vi "Begin.vi"(8 "error in":errorcluster) -> (0 "error out":errorcluster)   [LabVIEW 2018]
doc: "Called before other user functions, this VI is expected to open initial I/O refnums, load in file data, and do all program initialization. Notice that the <B>error out</B> terminal is simply used for data flow. Wiring it to other structures or subVIs ensures that this VI runs first."
uses:
  <vilib>/Rock Robotics/SystemInterfaces/DIO/FPGA_DIOPWMChannel.ctl
  <vilib>/Rock Robotics/WPI/SafetyOutput/WPI_SafetyOutputConfigMenu.ctl
  <vilib>/Rock Robotics/WPI/DriverStation/WPI_DriverStationRobotMode2.ctl
  <vilib>/Rock Robotics/WPI/Joystick/WPI_JoystickDeviceEnum.ctl
  <vilib>/Rock Robotics/WPI/Solenoid/WPI_SolenoidChannel.ctl
  <vilib>/Rock Robotics/WPI/Accelerometer/WPI_AccelerometerRange.ctl
  <vilib>/Rock Robotics/SystemInterfaces/DIO/FPGA_DIOChannel.ctl
  <vilib>/Rock Robotics/WPI/RobotDrive/WPI_RobotDriveOpen2MotorWithSPARK.vi
  Robot Global Data.vi
  <vilib>/Rock Robotics/Network Tables/NT Write String Array.vi
  <vilib>/Rock Robotics/WPI/Solenoid/WPI_SolenoidOpenSingle.vi
  <vilib>/Rock Robotics/WPI/Accelerometer/InternalAccelerometer/WPI_AccelerometerInternalOpen.vi
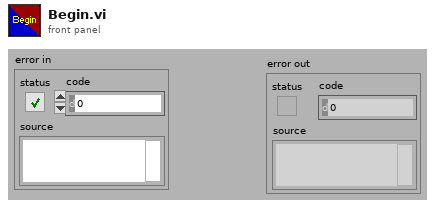
[diagram p1: front panel]
types:
  T1 = typedef "FPGA_DIOChannel.ctl" = enum8{"DIO 0", "DIO 1", "DIO 2", "DIO 3", "DIO 4", "DIO 5", "DIO 6", "DIO 7", "DIO 8", "DIO 9", "DIO MXP 0", "DIO MXP 1", "DIO MXP 2", "DIO MXP 3", "DIO MXP 4", "DIO MXP 5", "DIO MXP 6", "DIO MXP 7", "DIO MXP 8", "DIO MXP 9", "DIO MXP 10", "DIO MXP 11", "DIO MXP 12", "DIO MXP 13", "DIO MXP 14", "DIO MXP 15", "SPI Port CS1", "SPI Port CS2", "SPI Port CS3", "SPI Port MISO", "SPI Port MOSI", "Invalid"}
  T2 = typedef "WPI_SolenoidChannel.ctl" = enum8{"Solenoid 0", "Solenoid 1", "Solenoid 2", "Solenoid 3", "Solenoid 4", "Solenoid 5", "Solenoid 6", "Solenoid 7", "Invalid"}
  T3 = typedef "WPI_AccelerometerRange.ctl" = enum16{"+/- 2 g", "+/- 4 g", "+/- 8 g"}
  T4 = typedef "WPI_JoystickDeviceEnum.ctl" = enum16{"USB 0", "USB 1", "USB 2", "USB 3", "USB 4", "USB 5"}
  T5 = typedef "WPI_DriverStationRobotMode2.ctl" = enum16{"Autonomous Disabled", "Autonomous Enabled", "Teleop Disabled", "Teleop Enabled", "Disconnected", "Finish", "Test Disabled", "Test Enabled", "Emergency Stopped"}
  T6 = typedef "WPI_SafetyOutputConfigMenu.ctl" = enum16{"Enable", "Disable"}
  T7 = typedef "FPGA_DIOPWMChannel.ctl" = enum8{"PWM 0", "PWM 1", "PWM 2", "PWM 3", "PWM 4", "PWM 5", "PWM 6", "PWM 7", "PWM 8", "PWM 9", "PWM MXP 0", "PWM MXP 1", "PWM MXP 2", "PWM MXP 3", "PWM MXP 4", "PWM MXP 5", "PWM MXP 6", "PWM MXP 7", "PWM MXP 8", "PWM MXP 9", "Invalid"}
  T8 = typedef "WPI_JoystickDevRef.ctl" = cluster{"Device":T4}
  T9 = typedef "WPI_RobotDriveDevRef.ctl" = cluster{"DevStatus":errorcluster, "Motors[]":T10[], "Square Inputs":bool, "Max Output":dbl}
  T10 = typedef "WPI_MotorControlDeviceRef.ctl" = cluster{"DeviceStatus":errorcluster, "Type":T11, "PWM":cluster{"PWM Channel":T7, "DeadBand":T12}, "CAN":cluster{"Device Number":u8, "SetOutput VI Ref":variant, "GetOutput VI Ref":variant, "Enable VI Ref":variant, "Disable VI Ref":variant, "Data":variant}, "Invert":bool, "DIO PWM":cluster{"PWM \"Enable\" Channel":T7, "DIOChannel":T1, "PWM Rate":dbl}}
  T11 = typedef "WPI_MotorControlType.ctl" = enum16{"PWM", "CAN", "DIO PWM"}
  T12 = typedef "WPI_PWMDeadband.ctl" = cluster{"Name":string, "maxPositivePwm":i32, "minPositivePwm":i32, "centerPwm":i32, "maxNegativePwm":i32, "minNegativePwm":i32, "angularRange":u16}
  T13 = typedef "WPI_AccelerometerDevRef.ctl" = cluster{"DevStatus":errorcluster, "Scaling":T14, "Analog Channels":T15, "I2C Bus":T17, "SPI Bus":T18, "Accel Range":T19, "ADXL Axes":T20, "Handle":i32, "Device Address":u8, "Accel Type":enum16{"Analog", "ADXL345 I2C", "ADXL345 SPI", "Internal", "ADXL362 SPI"}}
  T14 = typedef "WPI_AccelerometerScaling.ctl" = cluster{"Gain (VoltsPerG)":dbl, "Center Voltage":dbl}
  T15 = typedef "WPI_AccelerometerAnalogChannels.ctl" = cluster{"X-Axis":T16, "Y-Axis":T16, "Z-Axis":T16}
  T16 = typedef "FPGA_AIChannel.ctl" = enum8{"AI 0", "AI 1", "AI 2", "AI 3", "AI MXP 0", "AI MXP 1", "AI MXP 2", "AI MXP 3", "Invalid"}
  T17 = typedef "i2c_bus.ctl" = enum16{"I2C On-Board", "I2C MXP", "Invalid"}
  T18 = typedef "spi_bus.ctl" = enum16{"SPI On-Board, CS0", "SPI On-Board, CS1", "SPI On-Board, CS2", "SPI On-Board, CS3", "SPI MXP", "Invalid"}
  T19 = typedef "ADXL345 Range.ctl" = u8
  T20 = typedef "WPI_AccelerometerADXL345 Axes.ctl" = cluster{"X-Axis":bool, "Y-Axis":bool, "Z-Axis":bool}
  T21 = typedef "WPI_SolenoidDevRef.ctl" = cluster{"DevStatus":errorcluster, "Pneumatics Control Module":u8, "Forward Solenoid Channel":T2, "Reverse Solenoid Channel":T2}
  T22 = typedef "WPI_AnalogChannelDevRef.ctl" = cluster{"DevStatus":errorcluster, "Analog Channel":T16}
  T23 = typedef "WPI_DigitalInputDevRef.ctl" = cluster{"DevStatus":errorcluster, "DIO Channel":T1}
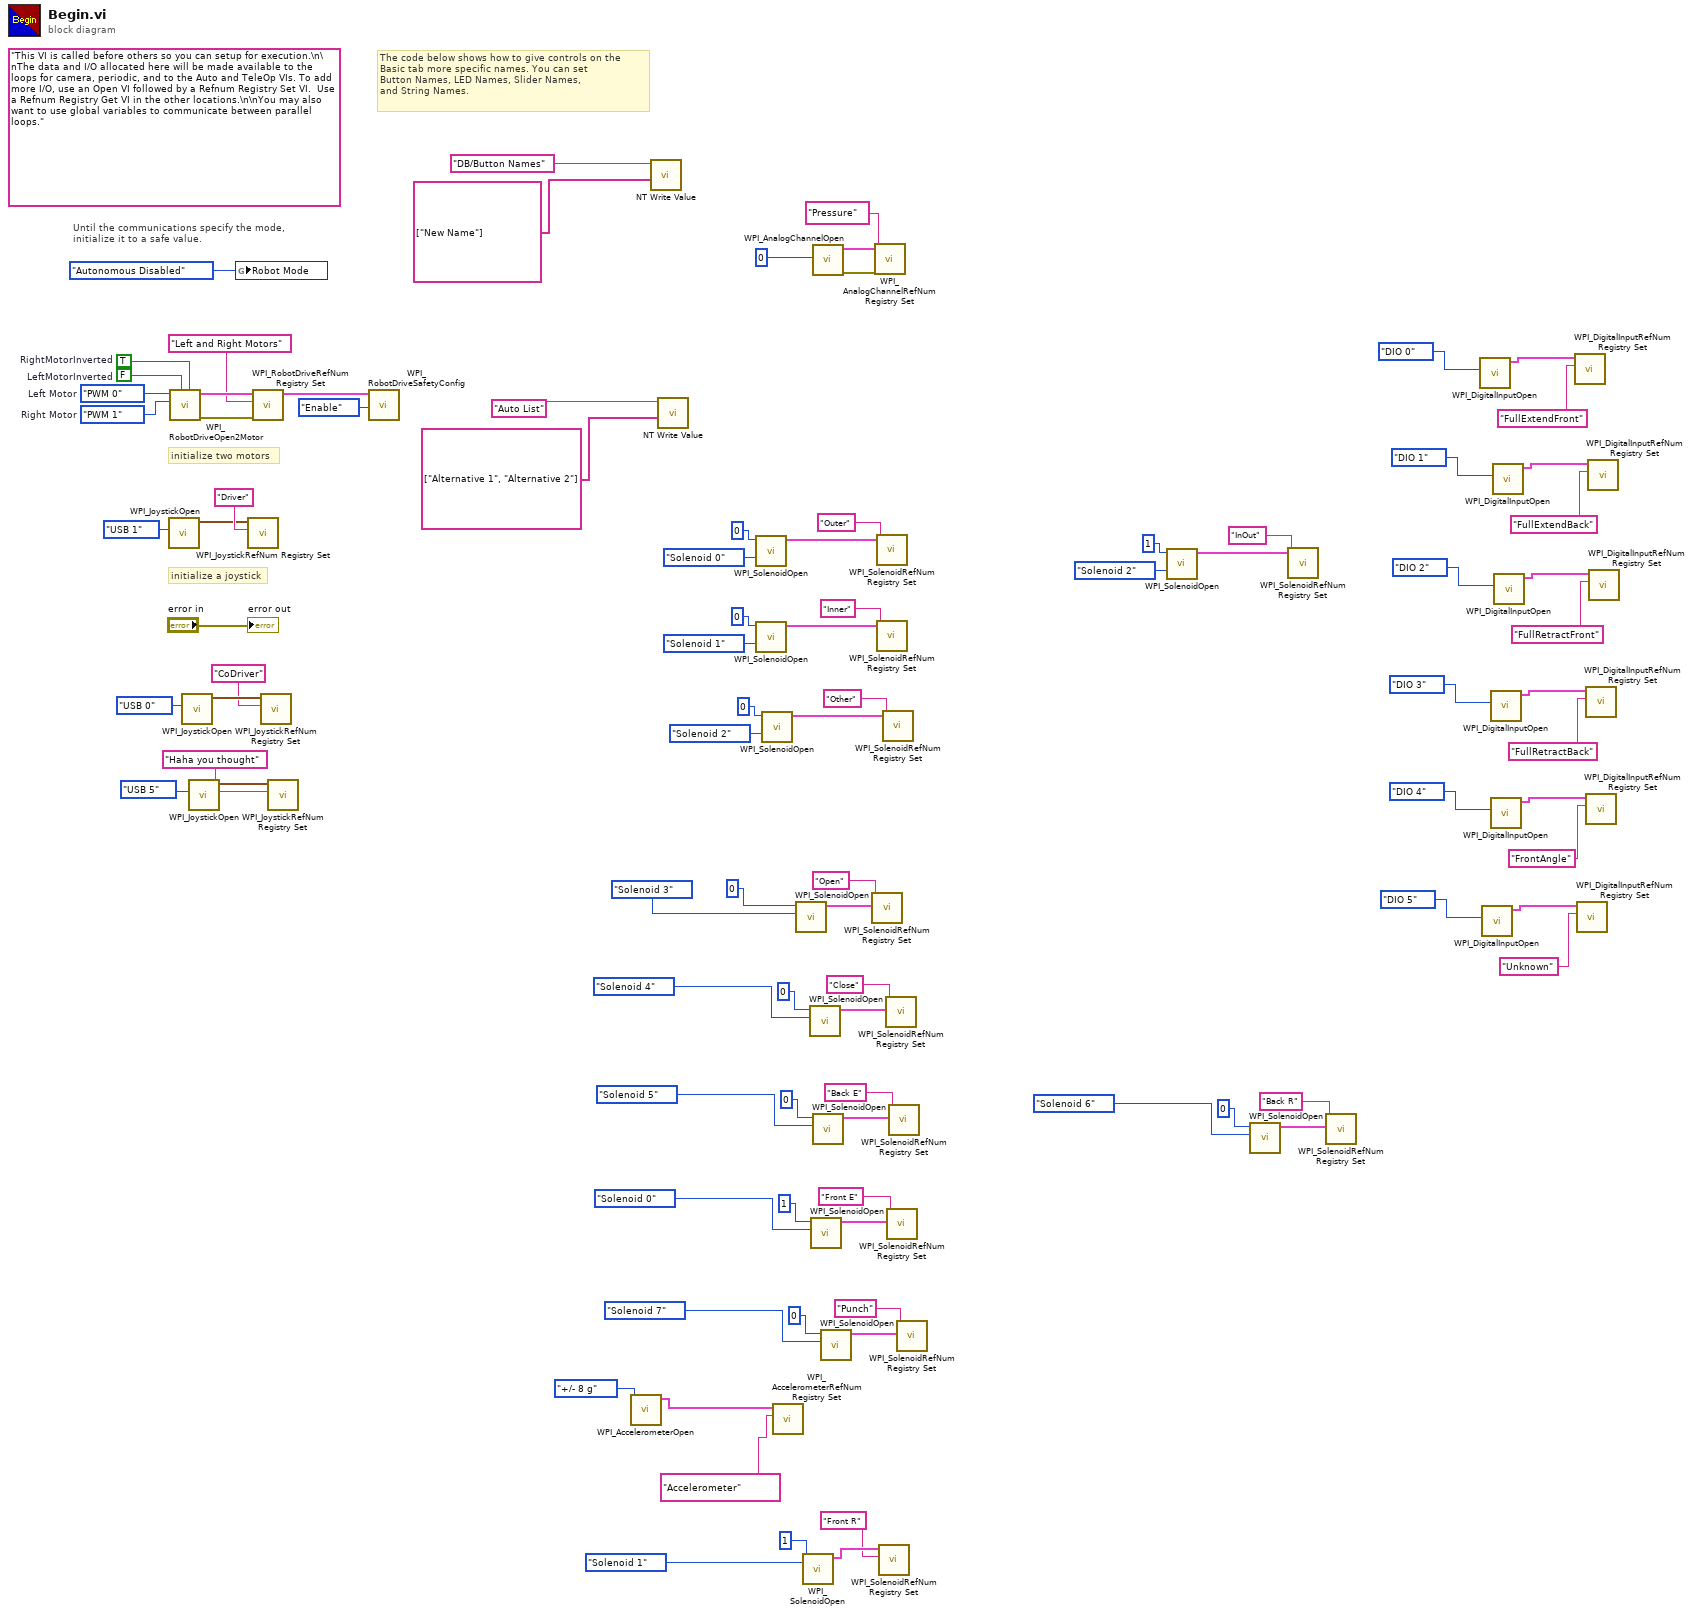
[diagram p0: block diagram]
diagram:
  (unwired) "This VI is called before others so you can setup for execution.\n\nThe data and I/O allocated here will be made available to the loops for camera, periodic, and to the Auto and TeleOp VIs. To add more I/O, use an Open VI followed by a Refnum Registry Set VI.  Use a Refnum Registry Get VI in the other locations.\n\nYou may also want to use global variables to communicate between parallel loops."
  w87 = FPGA_DIOPWMChannel."PWM 1"  # Right Motor
  w88 = FPGA_DIOPWMChannel."PWM 0"  # Left Motor
  w92 = FALSE  # LeftMotorInverted
  w93 = TRUE  # RightMotorInverted
  # "The code below shows how to give controls on the\nBasic tab more specific names. You can set\nButton Names, LED Names, Slider Names,\nand String Names."
  # "initialize a joystick"
  # "Until the communications specify the mode,\ninitialize it to a safe value."
  # "initialize two motors"
  n1 = call <vilib>:"WPI_JoystickOpen.vi"("JoystickDevice"=WPI_JoystickDeviceEnum."USB 1") -> ("JoystickDevRef"=w82:T8)  [unwired: 10 in]
  n2 = call-poly <vilib>:"WPI_RobotDriveOpen2Motor.vi"("Right Motor Inverted"=w93, "Left Motor Inverted"=w92, "Right Motor"=w87, "Left Motor"=w88) -> ("error out"=w89:errorcluster, "RobotDriveDevRef"=w91:T9)  [unwired: 1 in, 5 out]
  n3 = call <vilib>:"WPI_JoystickOpen.vi"("JoystickDevice"=WPI_JoystickDeviceEnum."USB 0") -> ("JoystickDevRef"=w58:T8)  [unwired: 10 in]
  n4 = call <vilib>:"WPI_JoystickOpen.vi"("JoystickDevice"=WPI_JoystickDeviceEnum."USB 5") -> ("JoystickDevRef"=w35:T8)  [unwired: 10 in]
  n5 = global write "Robot Global Data.vi" "Robot Mode"(WPI_DriverStationRobotMode2."Autonomous Disabled" ("Robot Mode")) -> ()
  n6 = call <vilib>:"WPI_JoystickRefNum Registry Set.vi"("refnum name"="Driver", "JoystickDevRef"=w82) -> ()  [unwired: 8 in, 2 out]
  n7 = call <vilib>:"WPI_RobotDriveRefNum Registry Set.vi"("error in (no error)"=w89, "refnum name"="Left and Right Motors", "RobotDriveDevRef"=w91) -> ("RobotDriveDevRef"=w86:T9)  [unwired: 1 in, 7 out]
  n8 = call <vilib>:"WPI_JoystickRefNum Registry Set.vi"("refnum name"="CoDriver", "JoystickDevRef"=w58) -> ()  [unwired: 8 in, 2 out]
  n9 = call <vilib>:"WPI_JoystickRefNum Registry Set.vi"("refnum name"="Haha you thought", "JoystickDevRef"=w35) -> ()  [unwired: 8 in, 2 out]
  n10 = call <vilib>:"WPI_RobotDriveSafetyConfig.vi"("mode"=WPI_SafetyOutputConfigMenu."Enable", "RobotDriveDevRef"=w86) -> ()  [unwired: 8 in, 2 out]
  n11 = call-poly <vilib>:"WPI_AccelerometerOpen.vi"("Accel Range"=WPI_AccelerometerRange."+/- 8 g") -> ("AccelerometerDevRef"=w32:T13)  [unwired: 9 in, 1 out]
  n12 = call-poly <vilib>:"NT Write Value.vi"("String Array"=string[] ["New Name"], "Name"="DB/Button Names") -> ()  [unwired: 9 in, 1 out]
  n13 = call-poly <vilib>:"NT Write Value.vi"("String Array"=string[] ["Alternative 1", "Alternative 2"], "Name"="Auto List") -> ()  [unwired: 9 in, 1 out]
  n14 = call-poly <vilib>:"WPI_SolenoidOpen.vi"("Solenoid Channel"=WPI_SolenoidChannel."Solenoid 0", "Pneumatics Control Module (0)"=u8 0) -> ("SolenoidDevRef"=w75:T21)  [unwired: 8 in, 1 out]
  n15 = call-poly <vilib>:"WPI_SolenoidOpen.vi"("Solenoid Channel"=WPI_SolenoidChannel."Solenoid 1", "Pneumatics Control Module (0)"=u8 0) -> ("SolenoidDevRef"=w64:T21)  [unwired: 8 in, 1 out]
  n16 = call-poly <vilib>:"WPI_SolenoidOpen.vi"("Solenoid Channel"=WPI_SolenoidChannel."Solenoid 2", "Pneumatics Control Module (0)"=u8 0) -> ("SolenoidDevRef"=w63:T21)  [unwired: 8 in, 1 out]
  n17 = call <vilib>:"WPI_AccelerometerRefNum Registry Set.vi"("refnum name"="Accelerometer", "AccelerometerDevRef"=w32) -> ()  [unwired: 8 in, 2 out]
  n18 = call-poly <vilib>:"WPI_SolenoidOpen.vi"("Solenoid Channel"=WPI_SolenoidChannel."Solenoid 3", "Pneumatics Control Module (0)"=u8 0) -> ("SolenoidDevRef"=w53:T21)  [unwired: 8 in, 1 out]
  n19 = call-poly <vilib>:"WPI_SolenoidOpen.vi"("Solenoid Channel"=WPI_SolenoidChannel."Solenoid 1" ("Reverse Solenoid Channel"), "Pneumatics Control Module (0)"=u8 1) -> ("SolenoidDevRef"=w28:T21)  [unwired: 8 in, 1 out]
  n20 = call-poly <vilib>:"WPI_SolenoidOpen.vi"("Solenoid Channel"=WPI_SolenoidChannel."Solenoid 4", "Pneumatics Control Module (0)"=u8 0) -> ("SolenoidDevRef"=w52:T21)  [unwired: 8 in, 1 out]
  n21 = call-poly <vilib>:"WPI_SolenoidOpen.vi"("Solenoid Channel"=WPI_SolenoidChannel."Solenoid 0", "Pneumatics Control Module (0)"=u8 1) -> ("SolenoidDevRef"=w44:T21)  [unwired: 8 in, 1 out]
  n22 = call <vilib>:"WPI_AnalogChannelOpen.vi"("Analog Channel"=0) -> ("error out"=w71:errorcluster, "AIDeviceRef"=w70:T22)  [unwired: 9 in]
  n23 = call-poly <vilib>:"WPI_SolenoidOpen.vi"("Solenoid Channel"=WPI_SolenoidChannel."Solenoid 5", "Pneumatics Control Module (0)"=u8 0) -> ("SolenoidDevRef"=w45:T21)  [unwired: 8 in, 1 out]
  n24 = call-poly <vilib>:"WPI_SolenoidOpen.vi"("Solenoid Channel"=WPI_SolenoidChannel."Solenoid 7", "Pneumatics Control Module (0)"=u8 0) -> ("SolenoidDevRef"=w37:T21)  [unwired: 8 in, 1 out]
  n25 = call <vilib>:"WPI_SolenoidRefNum Registry Set.vi"("refnum name"="Open", "SolenoidDevRef"=w53) -> ()  [unwired: 8 in, 2 out]
  n26 = call <vilib>:"WPI_AnalogChannelRefNum Registry Set.vi"("error in (no error)"=w71, "refnum name"="Pressure", "AIDeviceRef"=w70) -> ()  [unwired: 7 in, 2 out]
  n27 = call <vilib>:"WPI_SolenoidRefNum Registry Set.vi"("refnum name"="Outer", "SolenoidDevRef"=w75) -> ()  [unwired: 8 in, 2 out]
  n28 = call <vilib>:"WPI_SolenoidRefNum Registry Set.vi"("refnum name"="Inner", "SolenoidDevRef"=w64) -> ()  [unwired: 8 in, 2 out]
  n29 = call <vilib>:"WPI_SolenoidRefNum Registry Set.vi"("refnum name"="Front R", "SolenoidDevRef"=w28) -> ()  [unwired: 8 in, 2 out]
  n30 = call <vilib>:"WPI_SolenoidRefNum Registry Set.vi"("refnum name"="Other", "SolenoidDevRef"=w63) -> ()  [unwired: 8 in, 2 out]
  n31 = call <vilib>:"WPI_SolenoidRefNum Registry Set.vi"("refnum name"="Close", "SolenoidDevRef"=w52) -> ()  [unwired: 8 in, 2 out]
  n32 = call <vilib>:"WPI_SolenoidRefNum Registry Set.vi"("refnum name"="Front E", "SolenoidDevRef"=w44) -> ()  [unwired: 8 in, 2 out]
  n33 = call <vilib>:"WPI_SolenoidRefNum Registry Set.vi"("refnum name"="Back E", "SolenoidDevRef"=w45) -> ()  [unwired: 8 in, 2 out]
  n34 = call <vilib>:"WPI_SolenoidRefNum Registry Set.vi"("refnum name"="Punch", "SolenoidDevRef"=w37) -> ()  [unwired: 8 in, 2 out]
  n35 = call-poly <vilib>:"WPI_SolenoidOpen.vi"("Solenoid Channel"=WPI_SolenoidChannel."Solenoid 2", "Pneumatics Control Module (0)"=u8 1) -> ("SolenoidDevRef"=w19:T21)  [unwired: 8 in, 1 out]
  n36 = call-poly <vilib>:"WPI_SolenoidOpen.vi"("Solenoid Channel"=WPI_SolenoidChannel."Solenoid 6", "Pneumatics Control Module (0)"=u8 0) -> ("SolenoidDevRef"=w26:T21)  [unwired: 8 in, 1 out]
  n37 = call <vilib>:"WPI_SolenoidRefNum Registry Set.vi"("refnum name"="InOut", "SolenoidDevRef"=w19) -> ()  [unwired: 8 in, 2 out]
  n38 = call <vilib>:"WPI_SolenoidRefNum Registry Set.vi"("refnum name"="Back R", "SolenoidDevRef"=w26) -> ()  [unwired: 8 in, 2 out]
  n39 = call <vilib>:"WPI_DigitalInputOpen.vi"("DIO Channel"=FPGA_DIOChannel."DIO 0") -> ("DigitalInputDevRef"=w18:T23)  [unwired: 9 in, 1 out]
  n40 = call <vilib>:"WPI_DigitalInputOpen.vi"("DIO Channel"=FPGA_DIOChannel."DIO 5") -> ("DigitalInputDevRef"=w1:T23)  [unwired: 9 in, 1 out]
  n41 = call <vilib>:"WPI_DigitalInputOpen.vi"("DIO Channel"=FPGA_DIOChannel."DIO 3") -> ("DigitalInputDevRef"=w7:T23)  [unwired: 9 in, 1 out]
  n42 = call <vilib>:"WPI_DigitalInputOpen.vi"("DIO Channel"=FPGA_DIOChannel."DIO 4") -> ("DigitalInputDevRef"=w6:T23)  [unwired: 9 in, 1 out]
  n43 = call <vilib>:"WPI_DigitalInputOpen.vi"("DIO Channel"=FPGA_DIOChannel."DIO 1") -> ("DigitalInputDevRef"=w13:T23)  [unwired: 9 in, 1 out]
  n44 = call <vilib>:"WPI_DigitalInputOpen.vi"("DIO Channel"=FPGA_DIOChannel."DIO 2") -> ("DigitalInputDevRef"=w12:T23)  [unwired: 9 in, 1 out]
  n45 = call <vilib>:"WPI_DigitalInputRefNum Registry Set.vi"("refnum name"="FullExtendFront", "DigitalInputDevRef"=w18) -> ()  [unwired: 8 in, 2 out]
  n46 = call <vilib>:"WPI_DigitalInputRefNum Registry Set.vi"("refnum name"="Unknown", "DigitalInputDevRef"=w1) -> ()  [unwired: 8 in, 2 out]
  n47 = call <vilib>:"WPI_DigitalInputRefNum Registry Set.vi"("refnum name"="FullRetractBack", "DigitalInputDevRef"=w7) -> ()  [unwired: 8 in, 2 out]
  n48 = call <vilib>:"WPI_DigitalInputRefNum Registry Set.vi"("refnum name"="FrontAngle", "DigitalInputDevRef"=w6) -> ()  [unwired: 8 in, 2 out]
  n49 = call <vilib>:"WPI_DigitalInputRefNum Registry Set.vi"("refnum name"="FullExtendBack", "DigitalInputDevRef"=w13) -> ()  [unwired: 8 in, 2 out]
  n50 = call <vilib>:"WPI_DigitalInputRefNum Registry Set.vi"("refnum name"="FullRetractFront", "DigitalInputDevRef"=w12) -> ()  [unwired: 8 in, 2 out]
  "error out" <- "error in"
